vi "Signal Routing.vi"(10 "Boolean Array":bool[](array[boolean]), 11 "Data In":dynamicdata[](array[waveform])) -> (3 "Output":T1)   [LabVIEW 2022 SP3]
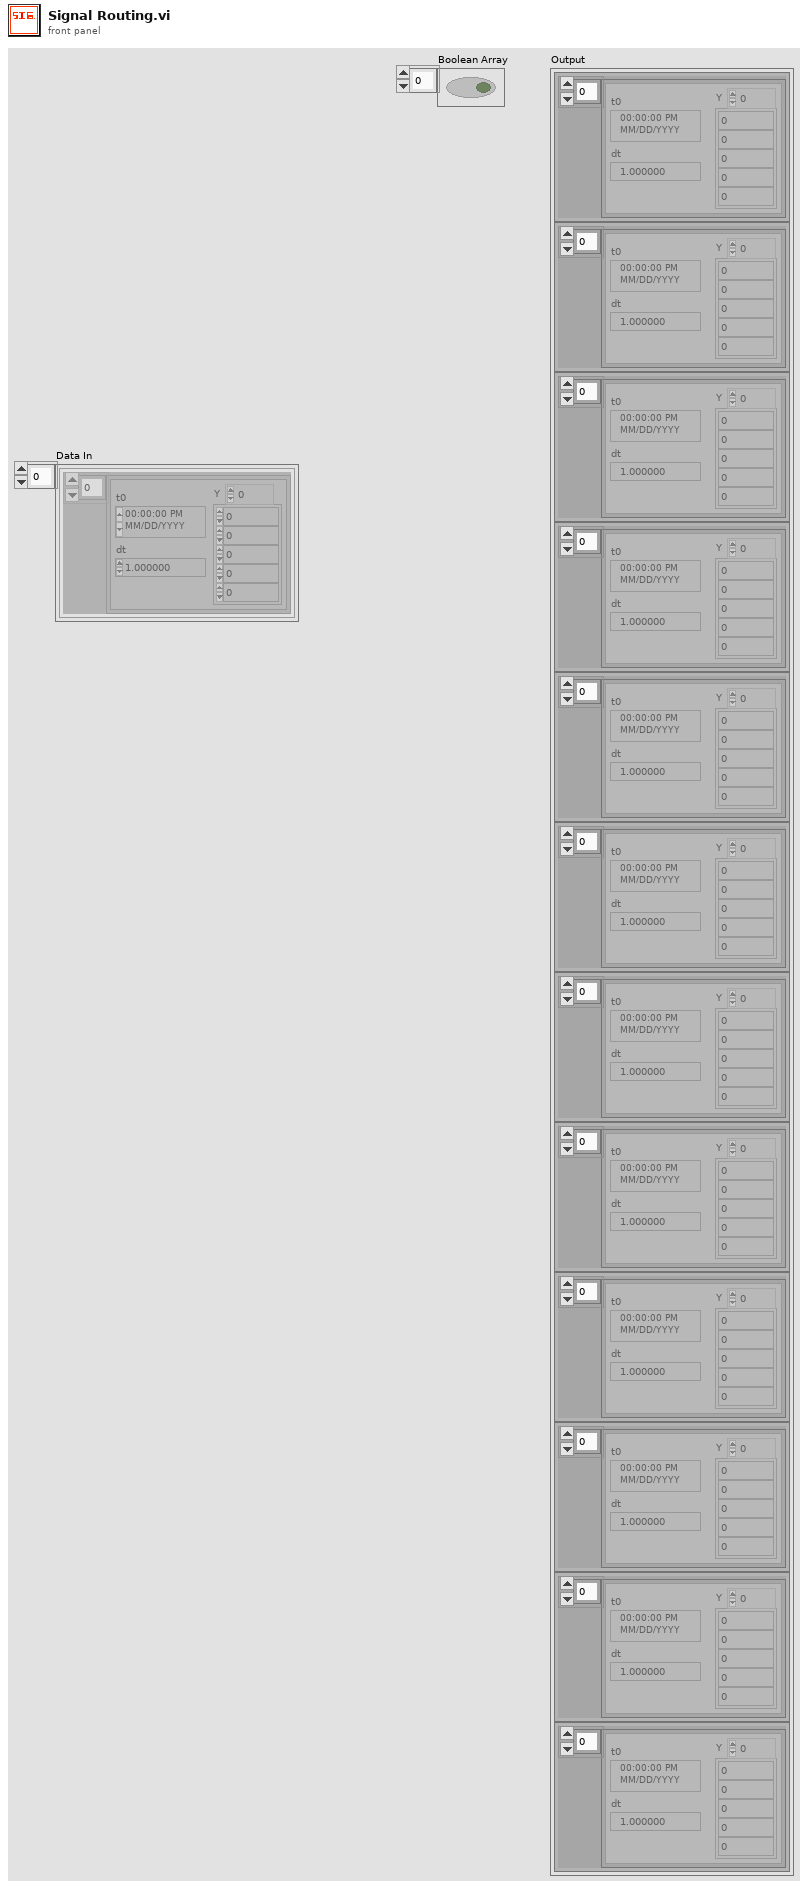
[diagram p1: front panel]
types:
  T1 = cluster{"Dynamic Data":dynamicdata, "Dynamic Data":dynamicdata, "Dynamic Data":dynamicdata, "Dynamic Data":dynamicdata, "Dynamic Data":dynamicdata, "Dynamic Data":dynamicdata, "Dynamic Data":dynamicdata, "Dynamic Data":dynamicdata, "Dynamic Data":dynamicdata, "Dynamic Data":dynamicdata, "Dynamic Data":dynamicdata, "Dynamic Data":dynamicdata}
  T2 = cluster{dynamicdata, dynamicdata, dynamicdata, dynamicdata, dynamicdata, dynamicdata, dynamicdata, dynamicdata, dynamicdata, dynamicdata, dynamicdata, dynamicdata}
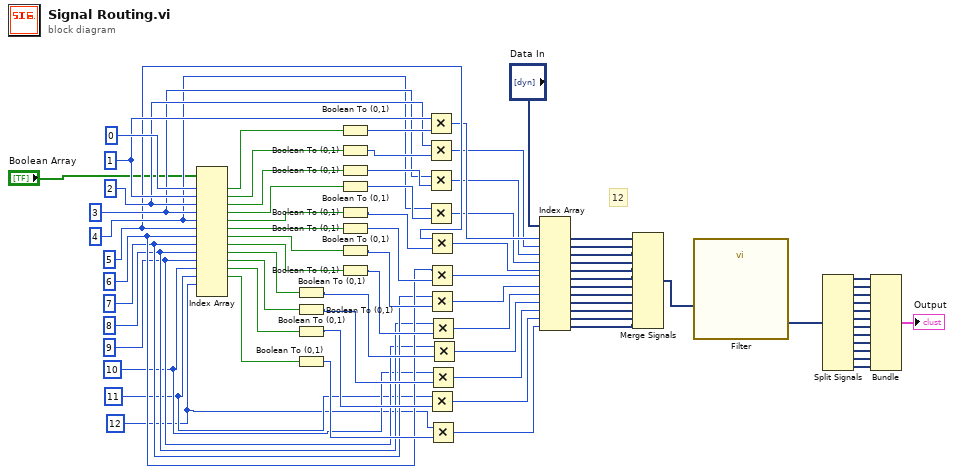
[diagram p0: block diagram]
diagram:
  w30 = 12 ("index")
  w31 = 11 ("index")
  w32 = 10 ("index")
  w33 = 9 ("index")
  w46 = 8 ("index")
  w47 = 7 ("index")
  w48 = 6 ("index")
  w49 = 5 ("index")
  w50 = 4 ("index")
  w51 = 3 ("index")
  w52 = 2 ("index")
  w53 = 1 ("index")
  # "12"
  n1 = Index Array(array="Boolean Array", index #1=0 ("index"), index #2=w53, index #3=w52, index #4=w51, index #5=w50, index #6=w49, index #7=w48, index #8=w47, index #9=w46, index #10=w33, index #11=w32, index #12=w31, index #13=w30) -> (element #1=w77:bool, element #2=w76:bool, element #3=w75:bool, element #4=w74:bool, element #5=w73:bool, element #6=w72:bool, element #7=w71:bool, element #8=w70:bool, element #9=w69:bool, element #10=w68:bool, element #11=w67:bool, element #12=w66:bool)  [unwired: 1 in, 2 out]
  n2 = Boolean To (0,1)(Boolean=w69) -> (0, 1=w57:i16)
  n3 = Boolean To (0,1)(Boolean=w68) -> (0, 1=w56:i16)
  n4 = Boolean To (0,1)(Boolean=w67) -> (0, 1=w55:i16)
  n5 = Boolean To (0,1)(Boolean=w66) -> (0, 1=w54:i16)
  n6 = Boolean To (0,1)(Boolean=w77) -> (0, 1=w65:i16)
  n7 = Boolean To (0,1)(Boolean=w76) -> (0, 1=w64:i16)
  n8 = Boolean To (0,1)(Boolean=w75) -> (0, 1=w63:i16)
  n9 = Boolean To (0,1)(Boolean=w74) -> (0, 1=w62:i16)
  n10 = Boolean To (0,1)(Boolean=w73) -> (0, 1=w61:i16)
  n11 = Boolean To (0,1)(Boolean=w72) -> (0, 1=w60:i16)
  n12 = Boolean To (0,1)(Boolean=w71) -> (0, 1=w59:i16)
  n13 = Boolean To (0,1)(Boolean=w70) -> (0, 1=w58:i16)
  n14 = Multiply(x=w53, y=w65) -> (x*y=w45:i32)
  n15 = Multiply(x=w52, y=w64) -> (x*y=w44:i32)
  n16 = Multiply(x=w51, y=w63) -> (x*y=w43:i32)
  n17 = Multiply(x=w50, y=w62) -> (x*y=w42:i32)
  n18 = Multiply(x=w49, y=w61) -> (x*y=w41:i32)
  n19 = Multiply(x=w48, y=w60) -> (x*y=w40:i32)
  n20 = Multiply(x=w47, y=w59) -> (x*y=w39:i32)
  n21 = Multiply(x=w31, y=w55) -> (x*y=w35:i32)
  n22 = Multiply(x=w46, y=w58) -> (x*y=w38:i32)
  n23 = Multiply(x=w32, y=w56) -> (x*y=w36:i32)
  n24 = Multiply(x=w30, y=w54) -> (x*y=w34:i32)
  n25 = Multiply(x=w33, y=w57) -> (x*y=w37:i32)
  n26 = Index Array(array="Data In", index #1=w45, index #2=w44, index #3=w43, index #4=w42, index #5=w41, index #6=w40, index #7=w39, index #8=w38, index #9=w37, index #10=w36, index #11=w35, index #12=w34) -> (element #1=w16:dynamicdata, element #2=w17:dynamicdata, element #3=w18:dynamicdata, element #4=w19:dynamicdata, element #5=w20:dynamicdata, element #6=w21:dynamicdata, element #7=w22:dynamicdata, element #8=w23:dynamicdata, element #9=w24:dynamicdata, element #10=w25:dynamicdata, element #11=w26:dynamicdata, element #12=w27:dynamicdata)
  n27 = Merge Signals(w16, w17, w18, w19, w20, w21, w22, w23, w24, w25, w26, w27) -> (w15:dynamicdata)
  n28 = call "Filter"("Signal"=w15) -> ("Filtered Signal"=w14:dynamicdata)  [unwired: 9 in, 1 out]
  n29 = Split Signals(w14) -> (w13:dynamicdata, w12:dynamicdata, w11:dynamicdata, w10:dynamicdata, w9:dynamicdata, w8:dynamicdata, w7:dynamicdata, w6:dynamicdata, w5:dynamicdata, w4:dynamicdata, w2:dynamicdata, w3:dynamicdata)  [unwired: 12 in]
  n30 = Bundle(w13, w12, w11, w10, w9, w8, w7, w6, w5, w4, w2, w3) -> (→"Output":T2)  [unwired: 1 in]
